vi "Online Order Waveform Extraction (DAQmx).vi"() -> ()   [LabVIEW 2023]
doc: "This example demonstrates how to apply an adaptive filter to online order waveform extraction. The vibration signal of a rotationary machine usually consists of vibration components from parts of the machine, such as gears and bearings. Order waveform extraction is to extract the vibration caused by a specific part from the overall vibration signal. This example uses the DAQmx VIs to acquire a vibration signal and an analog tachometer signal. This example then extracts the order waveforms continuously.\n\nComplete the following steps to use this example.\n\n1. Specify the <b>Tacho Channel</b>, <b>Vibration Channel</b> and <b>Sample Rate</b> for DAQ configuration.\n\n2. Specify the <b>Filter Length</b> and <b>Step Size</b> for the adaptive filter.\n\n3. Run the VI.\n\n4. Observe the <b>Vibration Signal</b> graph to compare the vibration signal and the order waveform.\n\n5. Change the <b>Order</b> value to observe the waveform at different orders."
uses:
  <vilib>/Platform/TimedLoop/XDataNode/timing_clust.ctl
  <vilib>/Platform/TimedLoop/XDataNode/nitl_modes.ctl
  <vilib>/Platform/TimedLoop/XDataNode/wakeup.ctl
  <vilib>/DAQmx/read.llb/DAQmx Read (Analog 2D DBL NChan NSamp).vi
  <vilib>/addons/Adaptive Filters/Create/AFT Create FIR Normalized LMS (Real).vi
  <vilib>/DAQmx/create/channels.llb/DAQmx Create Channel (AI-Voltage-Basic).vi
  <vilib>/DAQmx/configure/timing.llb/DAQmx Timing (Sample Clock).vi
  <vilib>/DAQmx/miscellaneous.llb/DAQmx Fill In Error Info.vi
  <vilib>/addons/Adaptive Filters/Processing/AFT Filter Signal and Update Coefficients (Real, PtByPt).vi
  <vilib>/Platform/TimedLoop/XDataNode/XDataNode.xnode
  <vilib>/Platform/TimedLoop/XDataNode/XDNodeRunTimeDep.lvlib
  <resource>/objmgr/daqmx.rc
  <vilib>/addons/Adaptive Filters/NI_AdaptiveFilter.lvlib
panel:
  in  "Vibration Channel":tag="Dev1/ai1"
  in  "Sample Rate (Hz)":dbl=25000.0
  in  "Reset":bool
  in  "Stop":bool
  in  "Filter Length":i32=64
  in  "Step Size":dbl=0.001
  in  "Order":dbl=1.0
  out "Vibration Signal":dbl[][](graph)
  out "Tachometer Signal":dbl[](graph)
  in  "Tacho Channel":tag="Dev1/ai0"
  # "Select Help>>Show Context Help and move the cursor over the VI icon of this example for more information."
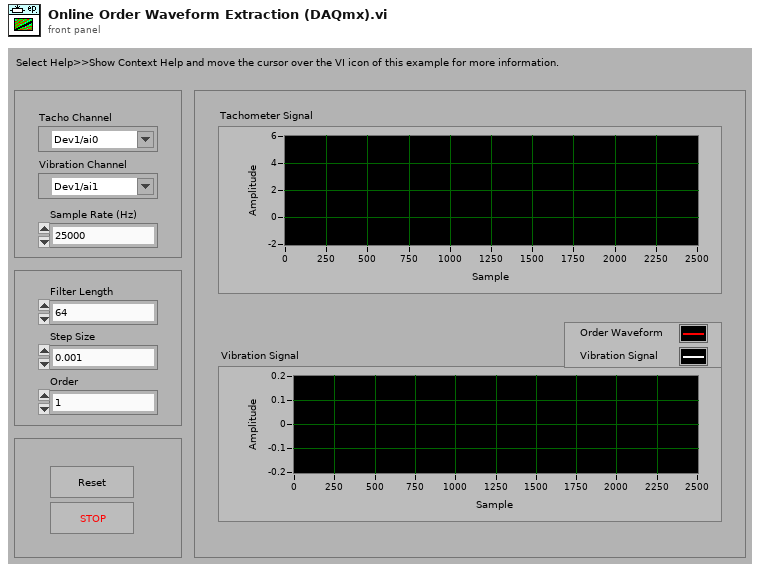
[diagram p1: front panel]
types:
  T1 = typedef "XDNodeRunTimeDep.lvlib/timing_clust.ctl" = cluster{"Expected End [f-1]":u64, "Actual End [f-1]":u64, "Finished Late? [f-1]":bool, "Expected End [i-1]":u64, "Actual End [i-1]":u64, "Finished Late? [i-1]":bool, "Expected Start [i]":u64, "Actual Start [i]":u64, "Expected Start [f]":u64, "Actual Start [f]":u64, "Source Name":string, "Structure Name":string, "Period":i64, "Deadline":i64, "Offset":i64, "Start":i64, "Priority":i32, "Timeout":i32, "Mode":T2, "Wakeup Reason":T3, "Error":errorcluster, "Source Type":string, "Secondary Source Type":string, "Global End Time":u64, "Global Start Time":u64, "Frame Duration":u64, "Iteration Duration":u64, "Assigned CPU":i32, "I/O Scan Engine Mode":u32}
  T2 = typedef "XDNodeRunTimeDep.lvlib/nitl_modes.ctl" = enum32{"No Change", "Process missed periods, maintain original phase", "Discard missed periods, maintain original phase", "Process missed periods, ignore original phase", "Discard missed periods, ignore original phase"}
  T3 = typedef "XDNodeRunTimeDep.lvlib/wakeup.ctl" = enum32{"Normal", "Aborted", "Asynchronous wakeup", "Timing source error", "Timed loop error", "Timeout"}
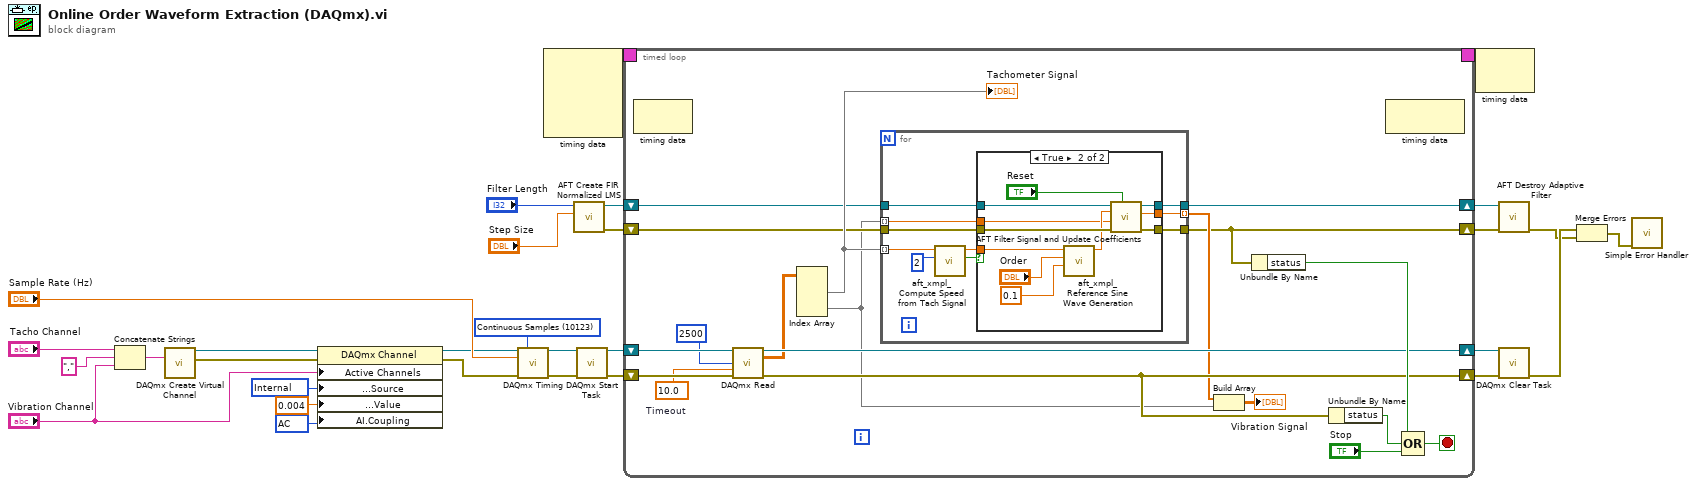
[diagram p0: block diagram]
diagram:
  w14 = 10045 items=["AC"=10045, "DC"=10050, "GND"=10066] ("AI.Coupling")
  w20 = 10200 items=["Internal"=10200, "External"=10167, "None"=10230] ("AI.Excit.Src")
  w30 = 10123 items=["Finite Samples"=10178, "Continuous Samples"=10123] ("sample mode")
  n1 = Concatenate Strings("Tacho Channel", "," ("string"), "Vibration Channel") -> (w5:string)
  n2 = call-poly <vilib>:"DAQmx Create Virtual Channel.vi"("physical channels"=w5) -> ("task out"=w16:refnum<k21>, "error out"=w15:errorcluster)  [unwired: 8 in, 5 out]
  n3 = property class="DAQmx Channel"(reference=w16, error in=w15, "Active Channels"="Vibration Channel", "Analog Input:General Properties:Signal Conditioning:Excitation:Source"=w20, "Analog Input:General Properties:Signal Conditioning:Excitation:Value"=0.004 ("AI.Excit.Val"), "AI.Coupling"=w14) -> (reference out=w18:refnum<k21>, error out=w17:errorcluster)
  n4 = call-poly <vilib>:"DAQmx Timing.vi"("task/channels in"=w18, "sample mode"=w30, "rate"="Sample Rate (Hz)", "error in"=w17) -> ("task out"=w29:refnum<k21>, "error out"=w28:errorcluster)  [unwired: 3 in, 7 out]
  n5 = node-c288() -> (w23:T1)  [unwired: 4 out]
  n6 = call-poly <vilib>:"AFT Create FIR Normalized LMS.vi"("step size"="Step Size", "filter length"="Filter Length") -> ("error out"=w10:errorcluster, "adaptive filter out"=w13:refnum<k20>)  [unwired: 2 in, 6 out]
  n7 = call <vilib>:"DAQmx Start Task.vi"("task/channels in"=w29, "error in"=w28) -> ("task out"=w27:refnum<k21>, "error out"=w26:errorcluster)  [unwired: 12 out]
  n8 = timed-loop {
    timing: w23 -> [_]
    timing-out: [_] -> w22
    shift-right: [w39] -> w12
    shift-left: w13 -> [w40]
    shift-right: [w33] -> w11
    shift-left: w10 -> [w38]
    shift-right: [w45] -> w25
    shift-left: w27 -> [w47]
    shift-right: [w48] -> w24
    shift-left: w26 -> [w46]
    stop <- w32 stop-if-true
    w44 = 10.0  # Timeout
    n9 = node-c288() -> ()  [unwired: 2 out]
    n10 = call-poly <vilib>:"DAQmx Read.vi"("task/channels in"=w47, "number of samples per channel"=2500, "timeout"=w44, "error in"=w46) -> ("task out"=w45:refnum<k21>, "data"=w43:dbl[][], "error out"=w48:errorcluster)  [unwired: 9 out]
    n11 = Index Array(array=w43) -> (element #1=w41:dbl[], element #2=w35:dbl[])  [unwired: 4 in]
    "Tachometer Signal" <- w41
    n12 = for {
      tunnel: w41 -> [w58] mode=indexing
      tunnel: w40 -> [w56]
      tunnel: w35 -> [w55] mode=indexing
      tunnel: [w54] -> w39
      tunnel: [w53] -> w33
      tunnel: w38 -> [w52]
      tunnel: [w51] -> w36 mode=indexing
      n13 = call "aft_xmpl_Compute Speed from Tach Signal.vi"("pulse/cycle"=2 ("Pulse/Cycle"), "Tach"=w58) -> ("Speed Available?"=w50:bool, "speed"=w57:dbl)  [unwired: 1 in, 7 out]
      n14 = case shown="True" w50 {
        tunnel: w57 -> [_ w66]
        tunnel: w56 -> [w61 w71]
        tunnel: w55 -> [_ w64]
        tunnel: [w61 w70] -> w54
        tunnel: [w60 w69] -> w53
        tunnel: w52 -> [w60 w68]
        tunnel: [_ w67] -> w51
        frame False {
        }
        frame True {
          n15 = call "aft_xmpl_Reference Sine Wave Generation.vi"("Amplitude"=0.1 ("Reference Amplitude"), "order"="Order", "Speed"=w66) -> ("Reference"=w65:dbl)  [unwired: 8 out]
          n16 = call-poly <vilib>:"AFT Filter Signal and Update Coefficients.vi"("reset? (F)"="Reset", "error in (no error)"=w68, "d(n)"=w64, "x(n)"=w65, "adaptive filter in"=w71) -> ("error out"=w69:errorcluster, "y(n)"=w67:dbl, "adaptive filter out"=w70:refnum<k20>)  [unwired: 1 in, 3 out]
        }
      }
    }
    n17 = Build Array(w36, w35) -> (→"Vibration Signal":dbl[][])
    n18 = Unbundle By Name(w33) -> ("status"=w49:bool)
    n19 = Unbundle By Name(w48) -> ("status"=w31:bool)
    n20 = node-c288() -> ()  [unwired: 2 out]
    n21 = Compound Arithmetic op=OR(w49, w31, "Stop") -> (w32:bool)
  }
  n22 = node-c288(w22) -> ()  [unwired: 1 out]
  n23 = call <vilib>:"AFT Destroy Adaptive Filter.vi"("error in (no error)"=w11, "adaptive filter in"=w12) -> ("error out"=w1:errorcluster)  [unwired: 9 out]
  n24 = call <vilib>:"DAQmx Clear Task.vi"("task in"=w25, "error in"=w24) -> ("error out"=w2:errorcluster)  [unwired: 13 out]
  n25 = Merge Errors(w2, w1) -> (w3:errorcluster)
  n26 = call <vilib>:"Simple Error Handler.vi"("error in (no error)"=w3) -> ()  [unwired: 1 in, 8 out]
